vi "Set port.vi"(8 "error in (no error)":errorcluster, 9 "Value":string, 10 "Puerto":dbl, 11 "Cypress in":refnum<class "Cypress.lvclass">) -> (0 "error out":errorcluster, 3 "Cypress out":refnum<class "Cypress.lvclass">)   [LabVIEW 2020, in "Cypress.lvclass"]
doc: "Override del papa Set Port"
uses:
  Cypress.lvclass
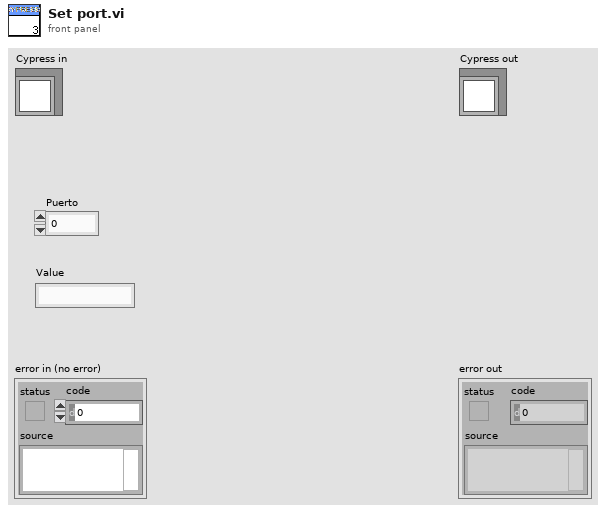
[diagram p1: front panel]
types:
  T1 = typedef "Serial Device.lvclass/serial device brand.ctl" = string
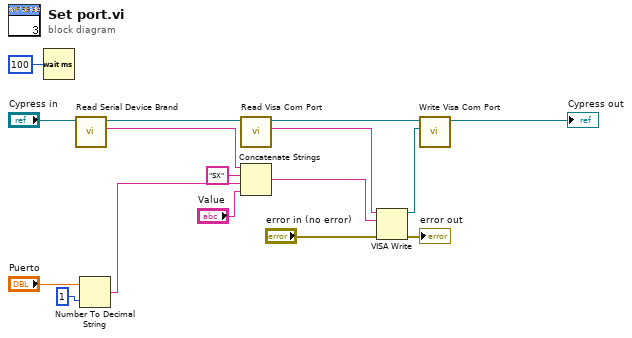
[diagram p0: block diagram]
diagram:
  n1 = Wait (ms)(milliseconds to wait=u32 100) -> ()  [unwired: 1 out]
  n2 = call-dynamic "Read Serial Device Brand.vi"("Serial Device in"="Cypress in") -> ("Serial Device Brand"=w12:T1, "Serial Device out"=w15:refnum<class "Cypress.lvclass">)  [unwired: 8 in, 1 out]
  n3 = Number To Decimal String(number="Puerto", width (-)=i16 1) -> (decimal integer string=w1:string)
  n4 = call-dynamic "Read Visa Com Port.vi"("Serial Device in"=w15) -> ("Visa Com Port"=w10:string, "Serial Device out"=w8:refnum<class "Cypress.lvclass">)  [unwired: 8 in, 1 out]
  n5 = Concatenate Strings(w12, "SX" ("string"), w1, "Value") -> (w6:string)
  n6 = VISA Write(VISA resource name=w10, write buffer=w6, error in (no error)="error in (no error)") -> (VISA resource name out=w9:refnum<visa-resource-name>, error out=→"error out":errorcluster)  [unwired: 1 out]
  n7 = call-dynamic "Write Visa Com Port.vi"("Visa Com Port"=w9, "Serial Device in"=w8) -> ("Serial Device out"=→"Cypress out":refnum<class "Cypress.lvclass">)  [unwired: 8 in, 1 out]
